vi "read_trajectory_frame.vi"(2 "Frame number":i32, 3 "error in":errorcluster, 4 "Ego pose":T2={"angular velocity"=[0.0, 0.0, 0.0], "velocity"=[0.0, 0.0, 0.0], "steering_direction"=0.0, "position"=[0.0, 0.0, 0.0], "orientation YPR"={"yaw"=0.001, "pitch"=0.0, "roll"=0.0}} {"orientation YPR"."yaw" min=0.0 step=0.1 format="%#_5f"; "steering_direction" format="%#_13g"}, 5 "simx in":T4={"Config"={"Trajectory"={"Number of frames"=0, "Frame number"=0, "Trajectory"=""}, "Weather"={"id"=""}}, "Connections"={"Simulator Connection"=refnum, "server_ip"="127.0.0.1", "Port"=0, "Sensor connections"=[]}, "Map"={"lanes"={"x"=[], "y"=[], "z"=[]}, "StartPosition"={"start_points"={"locations"=[], "rotations"=[], "type"=[]}, "StartRotation"=[], "StartLocation"=[]}, "Draw Map Size"={"Width"=0, "Height"=0}, "DrawArea"={"min_Y"=0.0, "min_X"=0.0, "Scale X"=0.0, "Scale Y"=0.0}, "Map"=bytes[0], "Map Geojson"=""}}) -> (0 "error out":errorcluster, 1 "Trajectory Frame String":string)   [LabVIEW 2019]
doc: "Modify the EGO pose with values given by the user on one frame of the given trajectory file."
uses:
  controls/simx_connection.ctl
  controls/config.ctl
  controls/trajectory.ctl
  controls/weather.ctl
  controls/connections.ctl
  controls/start_points.ctl
  <vilib>/Utility/miscctls.llb/LVBoundsTypeDef.ctl
panel:
  out "vehicles_format":T1(array[cluster])
  out "legacy_format":T3(array[cluster])
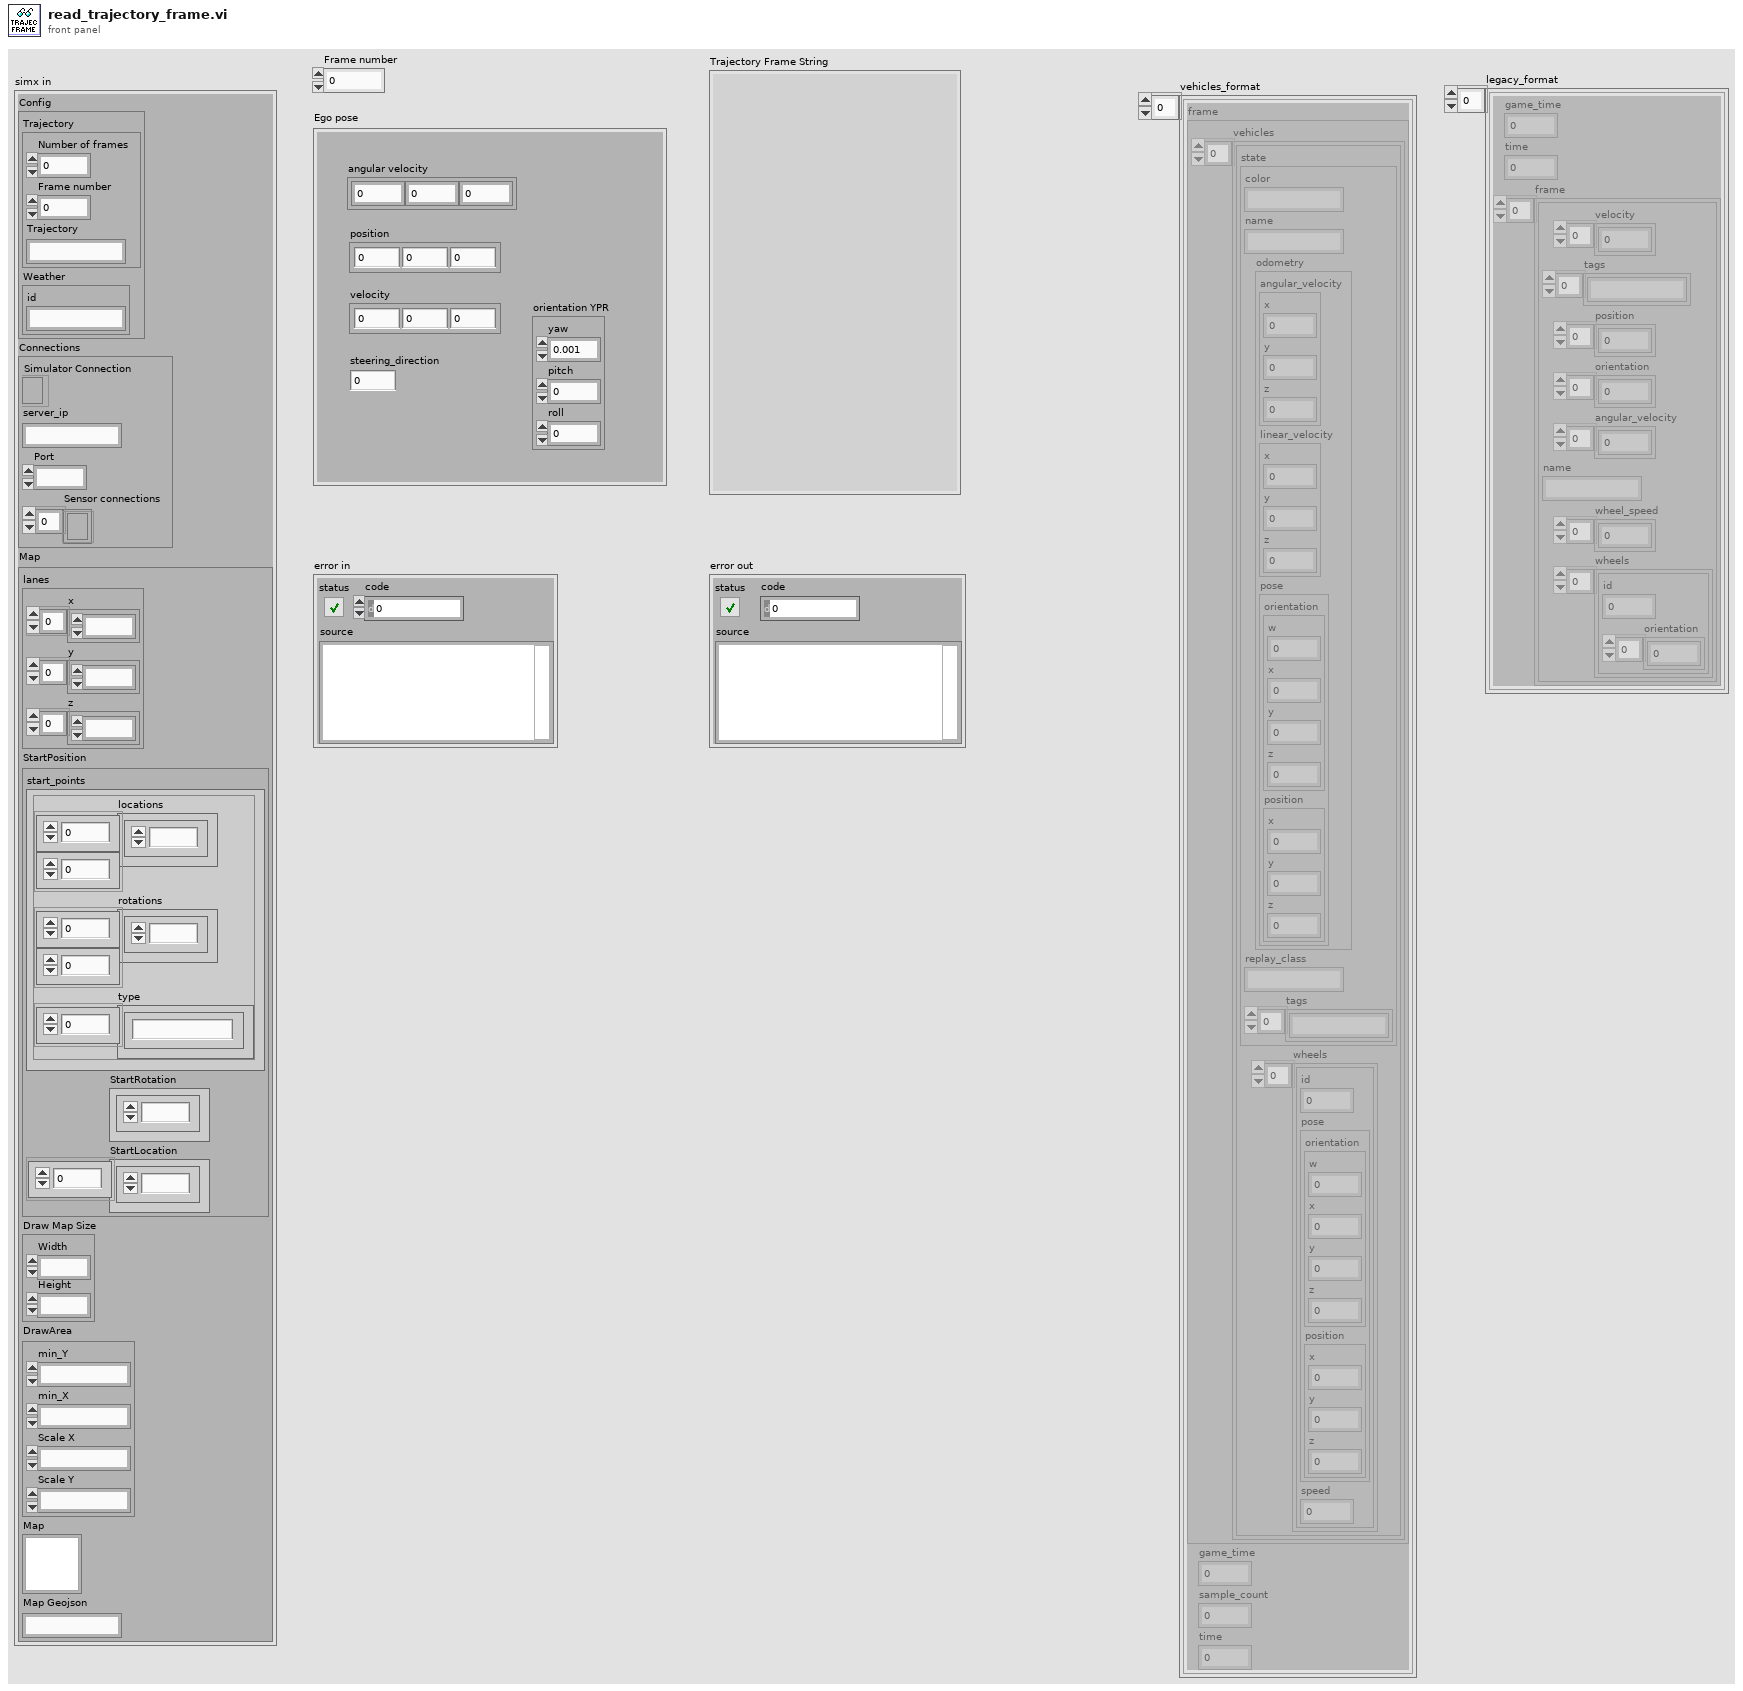
[diagram p1: front panel]
types:
  T1 = cluster{"frame":cluster{"vehicles":cluster{"state":cluster{"color":string, "name":string, "odometry":cluster{"angular_velocity":cluster{"x":i32, "y":i32, "z":dbl}, "linear_velocity":cluster{"x":i32, "y":i32, "z":dbl}, "pose":cluster{"orientation":cluster{"w":i32, "x":dbl, "y":i32, "z":i32}, "position":cluster{"x":i32, "y":i32, "z":i32}}}, "replay_class":string, "tags":string[]}, "wheels":cluster{"id":i32, "pose":cluster{"orientation":cluster{"w":dbl, "x":i32, "y":dbl, "z":i32}, "position":cluster{"x":dbl, "y":i32, "z":i32}}, "speed":i32}[]}[]}, "game_time":i32, "sample_count":i32, "time":i32}[]
  T2 = cluster{"angular velocity":dbl[], "velocity":dbl[], "steering_direction":dbl, "position":dbl[], "orientation YPR":cluster{"yaw":dbl, "pitch":dbl, "roll":dbl}}
  T3 = cluster{"game_time":dbl, "time":dbl, "frame":cluster{"velocity":dbl[], "tags":string[], "position":dbl[], "orientation":dbl[], "angular_velocity":dbl[], "name":string, "wheel_speed":dbl[], "wheels":cluster{"id":i32, "orientation":dbl[]}[]}[]}[]
  T4 = typedef "simx_connection.ctl" = cluster{"Config":T5, "Connections":T8, "Map":cluster{"lanes":cluster{"x":dbl[], "y":dbl[], "z":dbl[]}, "StartPosition":cluster{"start_points":T9, "StartRotation":dbl[], "StartLocation":dbl[]}, "Draw Map Size":T10, "DrawArea":cluster{"min_Y":dbl, "min_X":dbl, "Scale X":dbl, "Scale Y":dbl}, "Map":picture, "Map Geojson":string}}
  T5 = typedef "config.ctl" = cluster{"Trajectory":T6, "Weather":T7}
  T6 = typedef "trajectory.ctl" = cluster{"Number of frames":i32, "Frame number":i32, "Trajectory":string}
  T7 = typedef "weather.ctl" = cluster{"id":string}
  T8 = typedef "connections.ctl" = cluster{"Simulator Connection":refnum<k5>, "server_ip":string, "Port":i32, "Sensor connections":refnum<k5>[]}
  T9 = typedef "start_points.ctl" = cluster{"locations":dbl[][], "rotations":dbl[][], "type":string[]}
  T10 = typedef "LVBoundsTypeDef.ctl" = cluster{"Width":u32, "Height":u32}
  T11 = cluster{"frame":cluster{"vehicles":cluster{"state":cluster{"color":string, "name":string, "odometry":cluster{"angular_velocity":cluster{"x":dbl, "y":dbl, "z":dbl}, "linear_velocity":cluster{"x":dbl, "y":dbl, "z":dbl}, "pose":cluster{"orientation":cluster{"w":dbl, "x":dbl, "y":dbl, "z":dbl}, "position":cluster{"x":dbl, "y":dbl, "z":dbl}}}, "replay_class":string, "tags":string[]}, "wheels":cluster{"id":i32, "pose":cluster{"orientation":cluster{"w":dbl, "x":dbl, "y":dbl, "z":dbl}, "position":cluster{"x":dbl, "y":dbl, "z":dbl}}, "speed":dbl}[]}[]}, "game_time":dbl, "sample_count":dbl, "time":dbl}[]
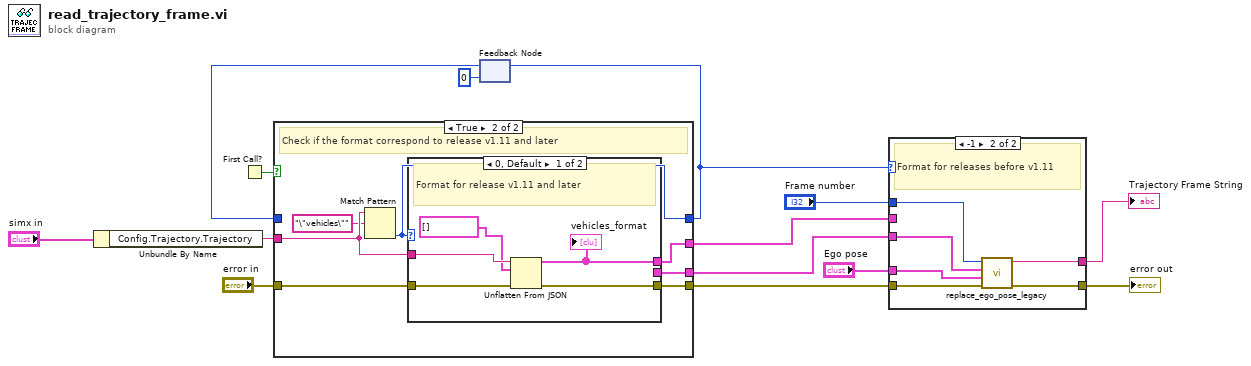
[diagram p0: block diagram]
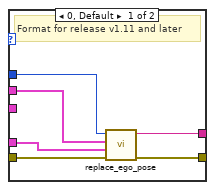
[diagram p2: hidden frame]
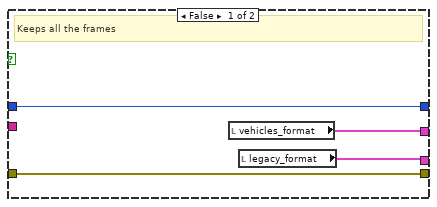
[diagram p3: hidden frame]
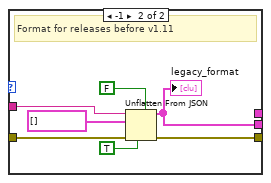
[diagram p4: hidden frame]
diagram:
  n1 = Unbundle By Name("simx in") -> ("Config.Trajectory.Trajectory"=w13:string)
  n2 = First Call?() -> (First Call?: T/F=w12:bool)
  n3 = feedback #1(0 ("offset past match")) -> (w2:i32)
  n4 = case shown="True" w12 {
    tunnel: w13 -> [_ w22]
    tunnel: [w18 w25] -> w10
    tunnel: "error in" -> [w17 w24]
    tunnel: [w17 w23] -> w8
    tunnel: [w16 w20] -> w4
    tunnel: [w15 w19] -> w3
    tunnel: w2 -> [w15 _]
    frame False {
      # "Keeps all the frames"
      n5 = local read "vehicles_format"() -> (w16:T1)
      n6 = local read "legacy_format"() -> (w18:T3)
    }
    frame True {
      # "Check if the format correspond to release v1.11 and later"
      n7 = Match Pattern(string=w22, regular expression="\"vehicles\"" ("search string")) -> (offset past match=w19:i32)  [unwired: 1 in, 3 out]
      n8 = case shown="0, Default" w19 {
        tunnel: w22 -> [w30 w37]
        tunnel: [_ w36] -> w25
        tunnel: w24 -> [w29 w34]
        tunnel: [w28 w33] -> w23
        tunnel: [w27 _] -> w20
        frame 0, Default {
          # "Format for release v1.11 and later"
          n9 = Unflatten From JSON(JSON string=w30, type and defaults=T11 [] ("value"), error in (no error)=w29) -> (value=w27:T11, error out=w28:errorcluster)  [unwired: 4 in]
          "vehicles_format" <- w27
        }
        frame -1 {
          # "Format for releases before v1.11"
          n10 = Unflatten From JSON(enable LabVIEW extensions? (T)=FALSE, JSON string=w37, type and defaults=T3 [], default null elements? (F)=TRUE, error in (no error)=w34) -> (value=w36:T3, error out=w33:errorcluster)  [unwired: 2 in]
          "legacy_format" <- w36
        }
      }
    }
  }
  n11 = feedback-in #1(w3) -> ()
  n12 = case shown="-1" w3 {
    tunnel: [w40 w49] -> w9
    tunnel: w10 -> [_ w48]
    tunnel: w8 -> [w41 w47]
    tunnel: "Frame number" -> [w43 w46]
    tunnel: [w39 w45] -> w6
    tunnel: "Ego pose" -> [w42 w44]
    tunnel: w4 -> [w38 _]
    frame 0, Default {
      # "Format for release v1.11 and later"
      n13 = call "replace_ego_pose.vi"("error in"=w41, "Ego pose"=w42, "Frames"=w38, "Frame number"=w43) -> ("error out"=w40:errorcluster, "Frame"=w39:string)  [unwired: 2 in]
    }
    frame -1 {
      # "Format for releases before v1.11"
      n14 = call "replace_ego_pose_legacy.vi"("error in"=w47, "Ego pose"=w44, "Frames"=w48, "Frame number"=w46) -> ("error out"=w49:errorcluster, "Frame"=w45:string)  [unwired: 2 in]
    }
  }
  "error out" <- w9
  "Trajectory Frame String" <- w6
